vi "Test HAL.vi"   [LabVIEW 2020]
uses:
  Abstract/Instrumento.lvclass
  Implemetations/Fuentes/Simulada/Simulada.lvclass
  C:/Users/enoea/Desktop/01 Queues User Events/HAL/Abstract/Instrumento.lvclass
  Implemetations/Fuentes/Instek/Instek.lvclass
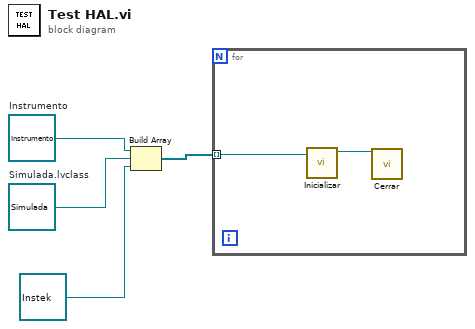
[diagram p0: block diagram]
diagram:
  w3 = refnum<class "Simulada.lvclass"> refnum  # Simulada.lvclass
  w4 = refnum<class "Instrumento.lvclass"> refnum  # Instrumento
  n1 = Build Array(w4, w3, refnum<class "Instek.lvclass"> refnum ("Instek.lvclass")) -> (w2:refnum<class "Instrumento.lvclass">[])
  n2 = for {
    tunnel: w2 -> [w6] mode=indexing
    n3 = call-dynamic "Inicializar.vi"("Instrumento in"=w6) -> ("Instrumento out"=w5:refnum<class "Instrumento.lvclass">)  [unwired: 9 in, 1 out]
    n4 = call-dynamic "Cerrar.vi"("Instrumento in"=w5) -> ()  [unwired: 9 in, 2 out]
  }
